vi "DCMotors_All.vi"(6 "Stop":bool, 8 "error in":errorcluster, 9 "Motors Renum":cluster{"Num":i32, "Directly":bool, "KM":dbl}[](array[cluster])=[{"Num"=1, "Directly"=TRUE, "KM"=0.97}, {"Num"=3, "Directly"=FALSE, "KM"=1.0}, {"Num"=0, "Directly"=FALSE, "KM"=0.98}, {"Num"=2, "Directly"=TRUE, "KM"=1.0}], 10 "Input":dbl[](array[slide])=[0.0, 0.0, -0.01, 0.0] step=1.0 scale=-100.0..100.0, 11 "CAN in":refnum<class "CAN.lvclass">) -> (0 "error out":errorcluster, 3 "CAN out":refnum<class "CAN.lvclass">)   [LabVIEW 2020]
uses:
  <vilib>/High Genius/HG_WSI_Tookit/Dependencies/Library/CAN/CAN.lvclass
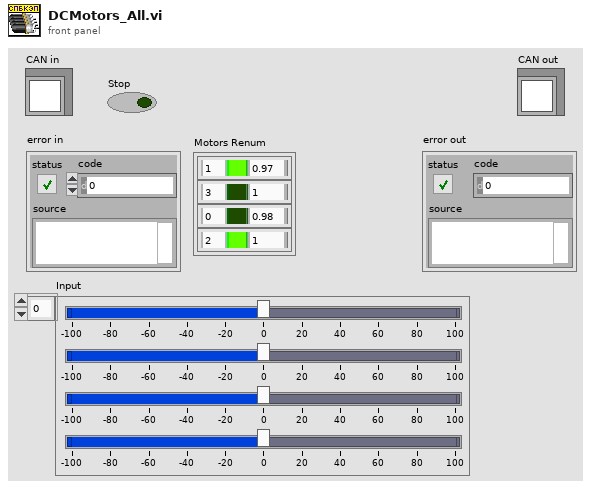
[diagram p1: front panel]
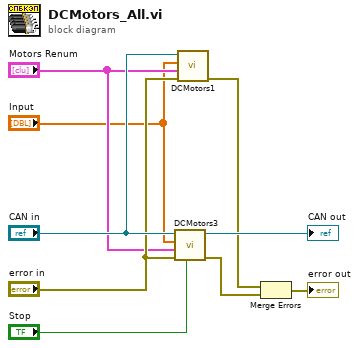
[diagram p0: block diagram]
diagram:
  n1 = call "DCMotors3.vi"("Stop"="Stop", "error in"="error in", "Motors Renum"="Motors Renum", "Input"="Input", "CAN in"="CAN in") -> ("error out"=w6:errorcluster, "CAN out"=→"CAN out":refnum<class "CAN.lvclass">)  [unwired: 5 in]
  n2 = call "DCMotors1.vi"("error in"="error in", "Motors Renum"="Motors Renum", "Input"="Input", "CAN in"="CAN in") -> ("error out"=w7:errorcluster)  [unwired: 6 in, 1 out]
  n3 = Merge Errors(w7, w6) -> (→"error out":errorcluster)
